vi "generateSimulatedData.vi"(8 "error in (no error)":errorcluster, 11 "ILCSimBasic in":refnum<class "ILCSimBasic.lvclass">) -> (0 "error out":errorcluster, 2 "stringRead":string, 3 "ILCSimBasic out":refnum<class "ILCSimBasic.lvclass">)   [LabVIEW 2013, in "ILCSimBasic.lvclass"]
uses:
  ILCSimBasic.lvclass
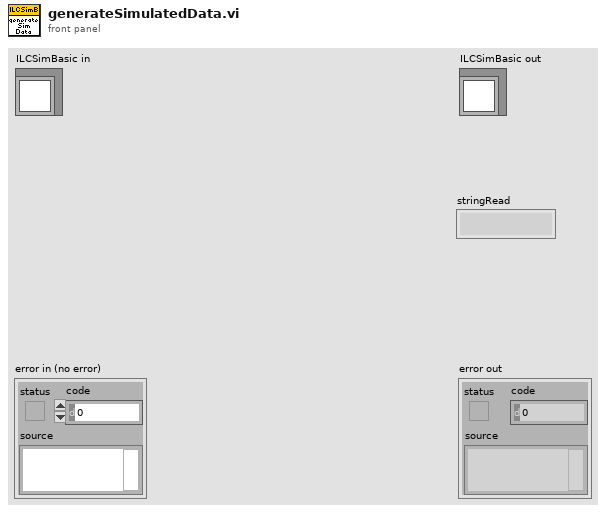
[diagram p1: front panel]
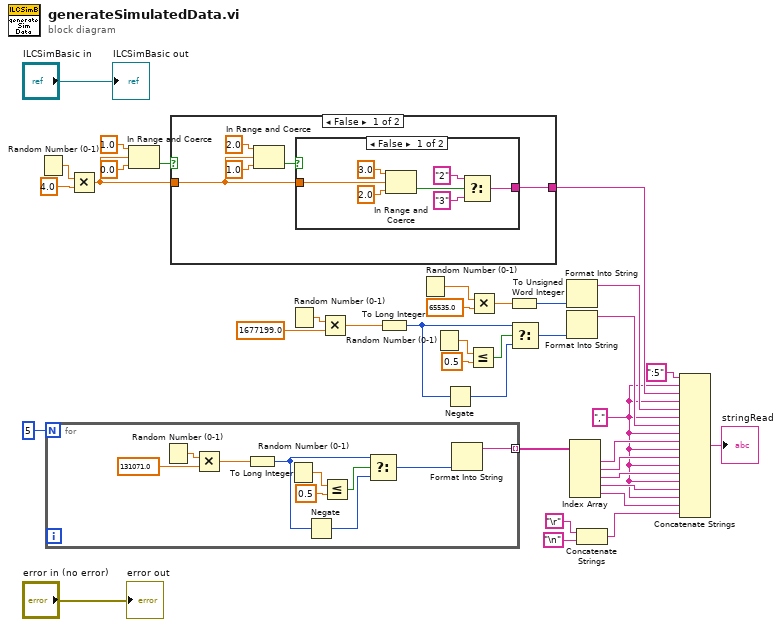
[diagram p0: block diagram]
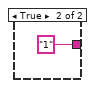
[diagram p2: hidden frame]
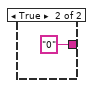
[diagram p3: hidden frame]
diagram:
  w11 = "," ("string")
  n1 = Random Number (0-1)() -> (number: 0 to 1=w6:dbl)
  n2 = for {
    N: 5 -> [_]
    tunnel: [w38] -> w16 mode=indexing
    n3 = Random Number (0-1)() -> (number: 0 to 1=w39:dbl)
    n4 = Multiply(x=w39, y=131071.0) -> (x*y=w43:dbl)
    n5 = To Long Integer(number=w43) -> (32bit integer=w44:i32)
    n6 = Random Number (0-1)() -> (number: 0 to 1=w41:dbl)
    n7 = Negate(x=w44) -> (-x=w46:i32)
    n8 = Less Or Equal?(x=w41, y=0.5) -> (x <= y?=w45:bool)
    n9 = Select(t=w44, s=w45, f=w46) -> (s? t:f=w47:i32)
    n10 = Format Into String(w47) -> (resulting string=w38:string)  [unwired: 3 in, 1 out]
  }
  n11 = Multiply(x=w6, y=4.0) -> (x*y=w1:dbl)
  n12 = In Range and Coerce(upper limit=1.0, x=w1, lower limit=0.0) -> (In Range?=w2:bool)  [unwired: 1 out]
  n13 = case shown="False" w2 {
    tunnel: [w49 "0" ("string")] -> w36
    tunnel: w1 -> [w48 _]
    frame False {
      n14 = In Range and Coerce(upper limit=2.0, x=w48, lower limit=1.0) -> (In Range?=w50:bool)  [unwired: 1 out]
      n15 = case shown="False" w50 {
        tunnel: [w54 "1" ("string")] -> w49
        tunnel: w48 -> [w53 _]
        frame False {
          n16 = In Range and Coerce(upper limit=3.0, x=w53, lower limit=2.0) -> (In Range?=w57:bool)  [unwired: 1 out]
          n17 = Select(t="2" ("string"), s=w57, f="3" ("string")) -> (s? t:f=w54:string)
        }
        frame True {
        }
      }
    }
    frame True {
    }
  }
  n18 = Random Number (0-1)() -> (number: 0 to 1=w30:dbl)
  n19 = Multiply(x=w30, y=1677199.0) -> (x*y=w26:dbl)
  n20 = To Long Integer(number=w26) -> (32bit integer=w25:i32)
  n21 = Random Number (0-1)() -> (number: 0 to 1=w34:dbl)
  n22 = Random Number (0-1)() -> (number: 0 to 1=w28:dbl)
  n23 = Negate(x=w25) -> (-x=w23:i32)
  n24 = Less Or Equal?(x=w28, y=0.5) -> (x <= y?=w24:bool)
  n25 = Multiply(x=w34, y=65535.0) -> (x*y=w33:dbl)
  n26 = To Unsigned Word Integer(number=w33) -> (unsigned 16bit integer=w32:u16)
  n27 = Select(t=w25, s=w24, f=w23) -> (s? t:f=w22:i32)
  n28 = Format Into String(w32) -> (resulting string=w31:string)  [unwired: 3 in, 1 out]
  n29 = Format Into String(w22) -> (resulting string=w21:string)  [unwired: 3 in, 1 out]
  n30 = Index Array(array=w16) -> (element #1=w15:string, element #2=w14:string, element #3=w13:string, element #4=w12:string, element #5=w10:string)  [unwired: 5 in]
  n31 = Concatenate Strings("\r", "\n") -> (w18:string)
  n32 = Concatenate Strings(":5" ("string"), w11, w36, w11, w31, w11, w21, w11, w15, w11, w14, w11, w13, w11, w12, w11, w10, w18) -> (→"stringRead":string)
  "error out" <- "error in (no error)"
  "ILCSimBasic out" <- "ILCSimBasic in"
